vi "Convert to JPEG String and Compress.vi"(10 "Image":T1(plugin-control)=refnum) -> (2 "JPEG Image String":string)   [LabVIEW 2023]
uses:
  <vilib>/vision/NI_Vision_Development_Module.lvlib
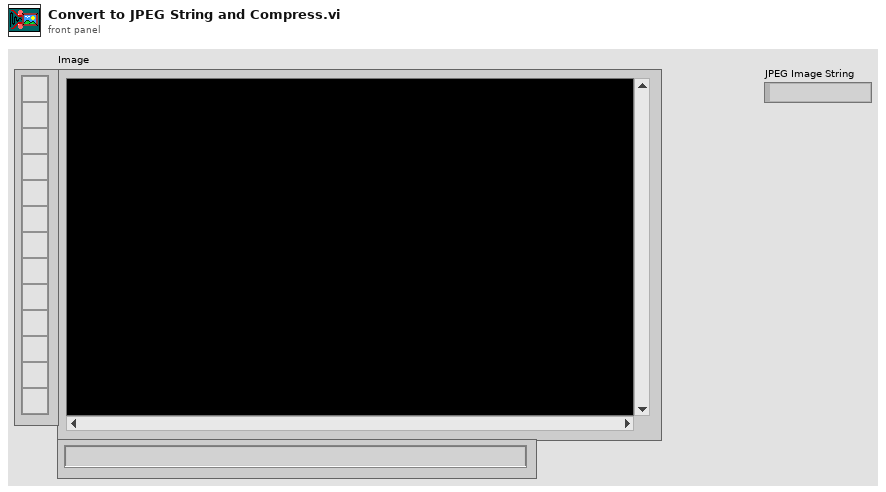
[diagram p1: front panel]
types:
  T1 = typedef "IMAQ Image.ctl" = refnum<image>
  T2 = typedef "Image Type" = u32
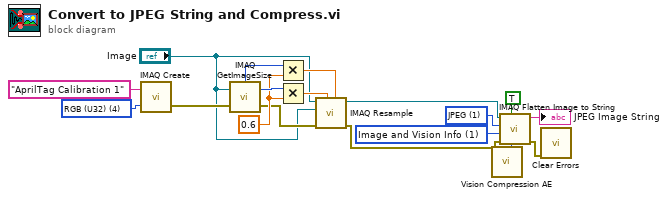
[diagram p0: block diagram]
diagram:
  w14 = T2 4 items=["Grayscale (U8)", "Grayscale (I16)", "Grayscale (SGL)", "Complex (CSG)", "RGB (U32)", "HSL (U32)", "RGB (U64)", "Grayscale (U16)"] ("Image Type")
  w10 = 0.6
  w17 = 1 items=["Image", "Image and Vision Info", "Reference to Image"] ("Type of Flatten (Image and Vision Info)")
  w18 = 1 items=["None", "JPEG", "PACKED BINARY"] ("Compression (None)")
  n1 = call "IMAQ Create"("Image Name"="AprilTag Calibration 1" ("string"), "Image Type"=w14) -> ("error out"=w4:errorcluster)  [unwired: 2 in, 2 out]
  n2 = call "IMAQ GetImageSize"("Image"="Image", "error in (no error)"=w4) -> ("Y Resolution"=w11:i32, "X Resolution"=w16:i32, "error out"=w8:errorcluster)  [unwired: 2 in]
  n3 = Multiply(x=w16, y=w10) -> (x*y=w12:dbl)
  n4 = Multiply(x=w11, y=w10) -> (x*y=w13:dbl)
  n5 = call "IMAQ Resample"("X Resolution"=w12, "Y Resolution"=w13, "error in (no error)"=w8, "Image Dst"="Image", "Image Src"="Image") -> ("error out"=w7:errorcluster, "Image Dst Out"=w2:T1)  [unwired: 5 in]
  n6 = call "Vision Compression AE.vi"() -> ("Compression"=w5:i32)  [unwired: 10 in, 1 out]
  n7 = call "IMAQ Flatten Image to String"("Quality (750)"=w5, "Flatten with Process-Unique Name (F)"=TRUE, "error in (no error)"=w7, "Type of Flatten (Image and Vision Info)"=w17, "Compression (None)"=w18, "Image"=w2) -> ("error out"=w6:errorcluster, "Data String"=→"JPEG Image String":string)  [unwired: 4 in]
  n8 = call <vilib>:"Clear Errors.vi"("error in (no error)"=w6) -> ()  [unwired: 5 in, 2 out]
